vi "save.vi"(6 "byte order (0:big-endian, network order)":T1(ring), 7 "prepend array or string size? (T)":bool, 8 "error in (no error)":errorcluster, 10 "file (use dialog)":path, 11 "PointCollection in":refnum<class "PointCollection.lvclass">) -> (0 "error out":errorcluster, 3 "PointCollection out":refnum<class "PointCollection.lvclass">)   [LabVIEW 2010, in "PointCollection.lvclass"]
uses:
  PointCollection.lvclass
  PointCollection.lvclass/PointCollection.ctl
panel:
  out "cancelled":bool
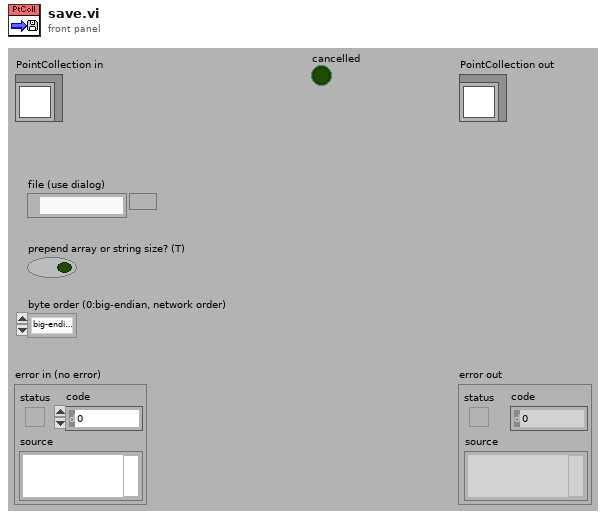
[diagram p1: front panel]
types:
  T1 = enum16{"big-endian, network order", "native, host order", "little-endian"}
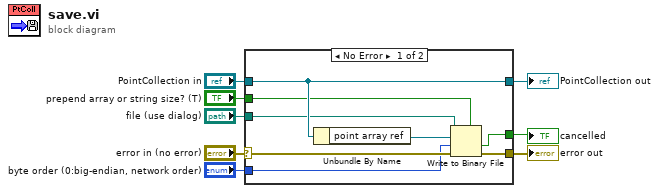
[diagram p0: block diagram]
diagram:
  n1 = case shown="No Error" "error in (no error)" {
    selector: "error in (no error)" -> [w14 w18]
    tunnel: [w13 w18] -> w7
    tunnel: [w16 w17] -> w5
    tunnel: "PointCollection in" -> [w16 w17]
    tunnel: "file (use dialog)" -> [w12 _]
    tunnel: "prepend array or string size? (T)" -> [w11 _]
    tunnel: [w10 _] -> w2
    tunnel: "byte order (0:big-endian, network order)" -> [w9 _]
    frame No Error {
      n2 = Unbundle By Name(w16) -> ("point array ref"=w15:refnum<data-value>)
      n3 = Write to Binary File(file (use dialog)=w12, data=w15, error in=w14, 5:w11, 9:w9) -> (cancelled=w10:bool, error out=w13:errorcluster)  [unwired: 1 in, 1 out]
    }
    frame Error {
    }
  }
  "error out" <- w7
  "PointCollection out" <- w5
  "cancelled" <- w2
